vi "EnergyStorage_Write Status.vi"(10 "EnergyStorage_Status":T1, 11 "EnergyStorage in":refnum<class "EnergyStorage.lvclass">) -> (3 "EnergyStorage out":refnum<class "EnergyStorage.lvclass">)   [LabVIEW 2015, in "EnergyStorage.lvclass"]
uses:
  EnergyStorage.lvclass
  EnergyStorage_Status.ctl
  EnergyStorage.lvclass/EnergyStorage.ctl
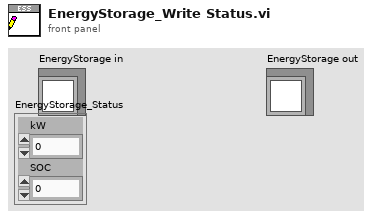
[diagram p1: front panel]
types:
  T1 = typedef "EnergyStorage.lvclass/EnergyStorage_Status.ctl" = cluster{"kW":dbl, "SOC":dbl}
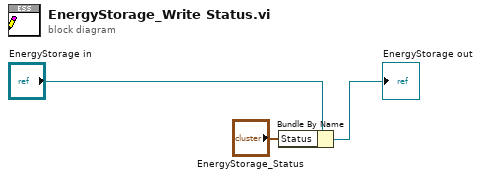
[diagram p0: block diagram]
diagram:
  n1 = Bundle By Name(cluster="EnergyStorage in", "Status"="EnergyStorage_Status") -> (→"EnergyStorage out":refnum<class "EnergyStorage.lvclass">)
